vi "Timer2.vi"(2 "Threshold":u32, 3 "Reset Timer":bool) -> (0 "Time (ms)":u32, 1 "Over Threshold?":bool)   [LabVIEW 2020]
doc: "This VI runs a relative millisecond timer. Setting Reset Timer to TRUE will reset the timer to 0 ms."
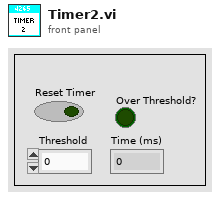
[diagram p1: front panel]
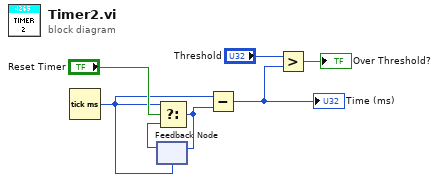
[diagram p0: block diagram]
diagram:
  n1 = Tick Count (ms)() -> (millisecond timer value=w5:u32)
  n2 = feedback #1(w5) -> (w4:u32)
  n3 = Select(t=w5, s="Reset Timer", f=w4) -> (s? t:f=w6:u32)
  n4 = feedback-in #1(w6) -> ()
  n5 = Subtract(x=w5, y=w6) -> (x-y=w3:u32)
  "Time (ms)" <- w3
  n6 = Greater?(x="Threshold", y=w3) -> (0:→"Over Threshold?":bool)
